vi "Write Name.vi"(10 "Name":string, 11 "((Pointer)) in":refnum<class "((Pointer)).lvclass">) -> (3 "((Pointer)) out":refnum<class "((Pointer)).lvclass">)   [LabVIEW 2016, in "((Pointer)).lvclass"]
uses:
  ((Pointer)).lvclass
  ((Pointer)).lvclass/((Pointer)).ctl
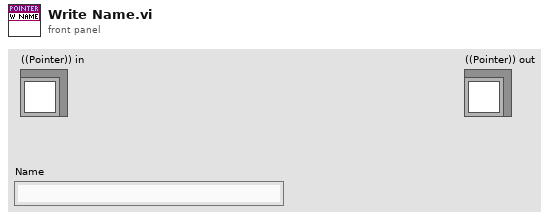
[diagram p1: front panel]
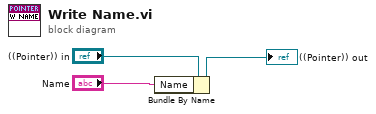
[diagram p0: block diagram]
diagram:
  n1 = Bundle By Name(cluster="((Pointer)) in", "Name"="Name") -> (→"((Pointer)) out":refnum<class "((Pointer)).lvclass">)
